vi "Connect to Artifactory (Config).vi"(5 "Artifactory in":refnum<class "Artifactory.lvclass">, 8 "error in (no error)":errorcluster, 10 "Config":T1={"username"="", "api-key"="", "server-uri"="", "repository-path"="", "auth-type"=enum."API Key"}, 11 "Local Repository":path) -> (0 "error out":errorcluster, 3 "Artifactory out":refnum<class "Artifactory.lvclass">)   [LabVIEW 2021, in "Artifactory.lvclass"]
uses:
  Artifactory.lvclass
  Config -- cluster.ctl
  Artifactory.lvclass/Artifactory.ctl
  <vilib>/LabVIEW Open Source Project/OpenSerializer.Base64/Base64_CharSet.vi
  auth-type -- enum.ctl
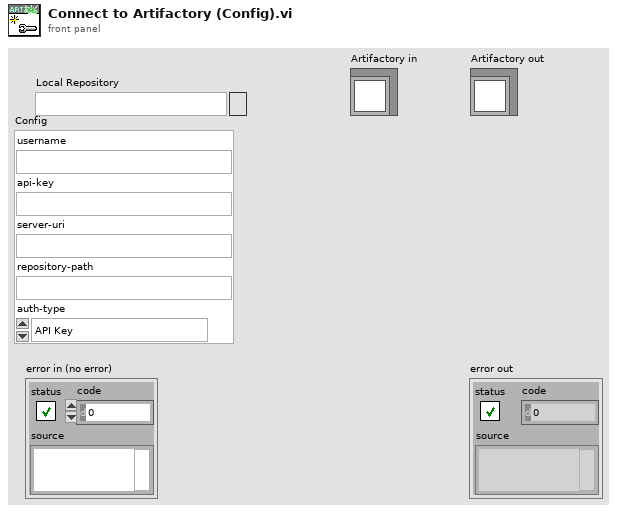
[diagram p1: front panel]
types:
  T1 = typedef "Artifactory.lvclass/Config -- cluster.ctl" = cluster{"username":string, "api-key":string, "server-uri":string, "repository-path":string, "auth-type":T2}
  T2 = typedef "Artifactory.lvclass/auth-type -- enum.ctl" = enum16{"Username + Password", "Username + API Key", "API Key", "Access token"}
  T3 = typedef "Artifactory.lvclass/Authorization -- cluster.ctl" = cluster{"auth-type":T2, "username":string, "api-key":string}
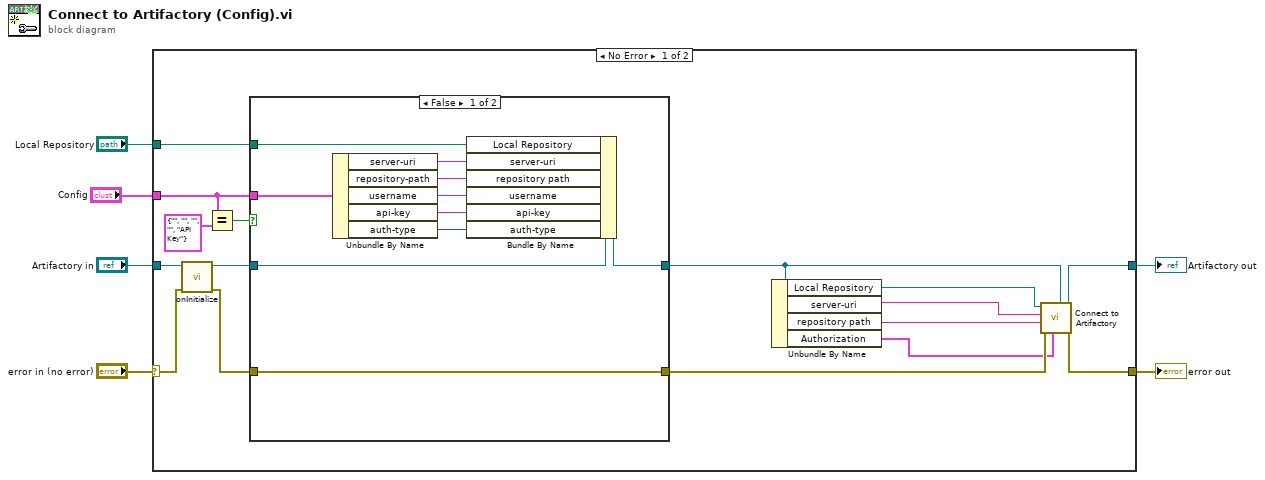
[diagram p0: block diagram]
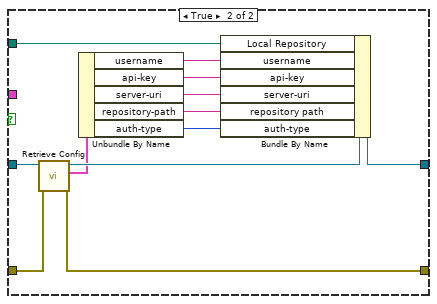
[diagram p2: hidden frame]
diagram:
  n1 = case shown="No Error" "error in (no error)" {
    selector: "error in (no error)" -> [w16 w46]
    tunnel: [w12 w46] -> w5
    tunnel: [w14 w45] -> w3
    tunnel: "Artifactory in" -> [w17 w45]
    tunnel: "Local Repository" -> [w22 _]
    tunnel: "Config" -> [w21 _]
    frame No Error {
      n2 = call-dynamic "onInitialize.vi"("error in (no error)"=w16, "Artifactory in"=w17) -> ("error out"=w15:errorcluster, "Artifactory out"=w18:refnum<class "Artifactory.lvclass">)  [unwired: 8 in]
      n3 = Equal?(x=w21, y=T1 {"username"="", "api-key"="", "server-uri"="", "repository-path"="", "auth-type"=enum."API Key"} ("Config")) -> (x = y?=w20:bool)
      n4 = case shown="False" w20 {
        tunnel: w22 -> [w32 w44]
        tunnel: [w31 w43] -> w11
        tunnel: w18 -> [w30 w42]
        tunnel: w21 -> [w28 _]
        tunnel: [w29 w39] -> w13
        tunnel: w15 -> [w29 w40]
        frame False {
          n5 = Unbundle By Name(w28) -> ("server-uri"=w27:string, "repository-path"=w26:string, "username"=w25:string, "api-key"=w24:string, "auth-type"=w23:T2)
          n6 = Bundle By Name(cluster=w30, "Local Repository"=w32, "server-uri"=w27, "repository path"=w26, "username"=w25, "api-key"=w24, "auth-type"=w23) -> (w31:refnum<class "Artifactory.lvclass">)
        }
        frame True {
          n7 = call-dynamic "Retrieve Config.vi"("error in"=w40, "Artifactory"=w42) -> ("error out"=w39:errorcluster, "Config"=w38:T1, "Artifactory out"=w41:refnum<class "Artifactory.lvclass">)  [unwired: 6 in, 1 out]
          n8 = Unbundle By Name(w38) -> ("username"=w34:string, "api-key"=w35:string, "server-uri"=w36:string, "repository-path"=w37:string, "auth-type"=w33:T2)
          n9 = Bundle By Name(cluster=w41, "Local Repository"=w44, "username"=w34, "api-key"=w35, "server-uri"=w36, "repository path"=w37, "auth-type"=w33) -> (w43:refnum<class "Artifactory.lvclass">)
        }
      }
      n10 = Unbundle By Name(w11) -> ("Local Repository"=w10:path, "server-uri"=w9:string, "repository path"=w8:string, "Authorization"=w7:T3)
      n11 = call "Connect to Artifactory.vi"("Artifactory in"=w11, "Authorization"=w7, "error in (no error)"=w13, "repository path"=w8, "server-uri"=w9, "Local Repository"=w10) -> ("error out"=w12:errorcluster, "Artifactory out"=w14:refnum<class "Artifactory.lvclass">)  [unwired: 4 in]
    }
    frame Error {
    }
  }
  "error out" <- w5
  "Artifactory out" <- w3
